vi "PH_Beamline.set Force Sensor State in GUI.vi"(0 "i ref in":refnum<vi>, 1 "Force Sensor GUI Ref":refnum<vi>, 3 "Subscriber State":T1 items=["no info", "off/false/out", "on/true/in", "Failure", "Alarm", "Status 1", "Status 2", "Status 3"], 4 "No Link":bool, 5 "error in (no error)":errorcluster) -> (14 "i ref out":refnum<vi>, 19 "error out":errorcluster)   [LabVIEW 2014, in "PH_Beamline.lvlib"]
doc: "This VI writes the incoming information about a Force Sensor to the GUI."
uses:
  PH_Beamline.lvlib
  PH_StatusHandler/PH_StatusHandler.Status.ctl
  PH_Common/PH_Common.lvlib
  PH_StatusHandler/PH_StatusHandler.lvlib
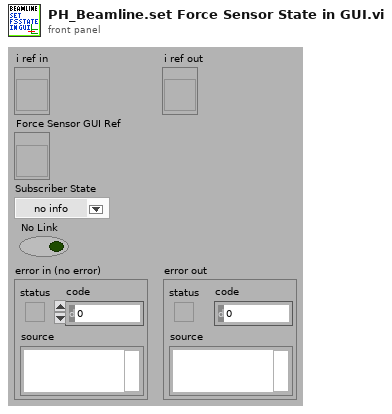
[diagram p1: front panel]
types:
  T1 = typedef "PH_StatusHandler.lvlib/PH_StatusHandler.Status.ctl" = i16
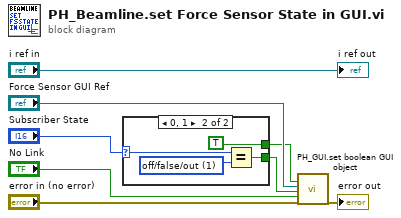
[diagram p0: block diagram]
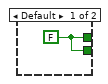
[diagram p2: hidden frame]
diagram:
  n1 = case shown="0, 1" "Subscriber State" {
    selector: "Subscriber State" -> [_ w12]
    tunnel: [w9 TRUE] -> w2
    tunnel: [w9 w10] -> w1
    frame Default {
      w9 = FALSE
    }
    frame 0, 1 {
      w11 = T1 1 items=["no info", "off/false/out", "on/true/in", "Failure", "Alarm", "Status 1", "Status 2", "Status 3"] ("y")
      n2 = Equal?(x=w12, y=w11) -> (x = y?=w10:bool)
    }
  }
  n3 = call "PH_GUI.set boolean GUI object.vi"("Visible (true)"=w2, "Boolean Knob GUI Ref"="Force Sensor GUI Ref", "Value"=w1, "Blinking? (false)"="No Link", "error in (no error)"="error in (no error)") -> ("error out"=→"error out":errorcluster)  [unwired: 14 in]
  "i ref out" <- "i ref in"
